vi "DUT_Handler_Simple_SoftFP.vi"(0 "reference in":refnum<class "DUT_Handler_Simple.lvclass">, 2 "Floating":bool, 5 "error in (no error)":errorcluster) -> (14 "reference out":refnum<class "DUT_Handler_Simple.lvclass">, 19 "error out":errorcluster)   [LabVIEW 2022 SP3, in "DUT_Handler_Simple.lvlib" / "DUT_Handler_Simple.lvclass"]
uses:
  DUT_Handler_Simple.lvclass
  Components/DUT_Handler_Base.lvlibp/EventData.ctl
  Components/ViPER.lvlibp/ViPER.lvclass
  C:/Projects/Medulla/ViPER/Examples/Flux_Capacitor_Tester/Components/ViPER.lvlibp/ViPER.lvclass
  Components/DUT_Handler_Base.lvlibp/DUT_Handler_Base.lvclass
panel:
  in  "Enable":bool
  in  "Load":bool
  out "event_data":T1={"Action"=enum."MoveIn", "SN"="", "BN"="", "DUT__ID"=0, "Message"="", "From"="", "To"=""}
  out "Enabled":bool
  in  "Move To":string
  in  "Move Out":bool
  in  "Move In":bool
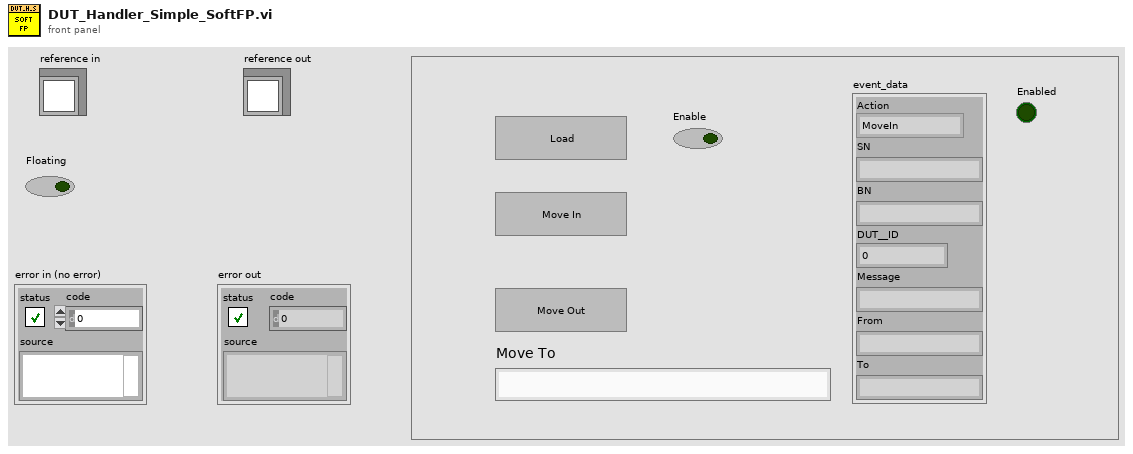
[diagram p1: front panel]
types:
  T1 = typedef "DUT_Handler_Base.lvlibp/DUT_Handler_Base.lvclass/EventData.ctl" = cluster{"Action":enum16{"Load", "Cancel", "MoveIn", "MoveOut", "Abort", "Msg", "Enabled", "Disabled", "Fault", "Shutdown"}, "SN":string, "BN":string, "DUT__ID":u32, "Message":string, "From":string, "To":string}
  T2 = enum32{"Invalid", "Standard", "Closed", "Hidden", "Minimized", "Maximized"}
  T3 = typedef "DUT_Handler_Simple.lvlib/DUT_Handler_Simple.lvclass/ObjectAttributes.ctl" = cluster{"Config":T4, "event_data":T1, "Enabled":bool, "Barcode_Reader":refnum<class "Barcode_Reader_Base.lvclass">}
  T4 = typedef "DUT_Handler_Simple.lvlib/DUT_Handler_Simple.lvclass/Config.ctl" = cluster{"default":string}
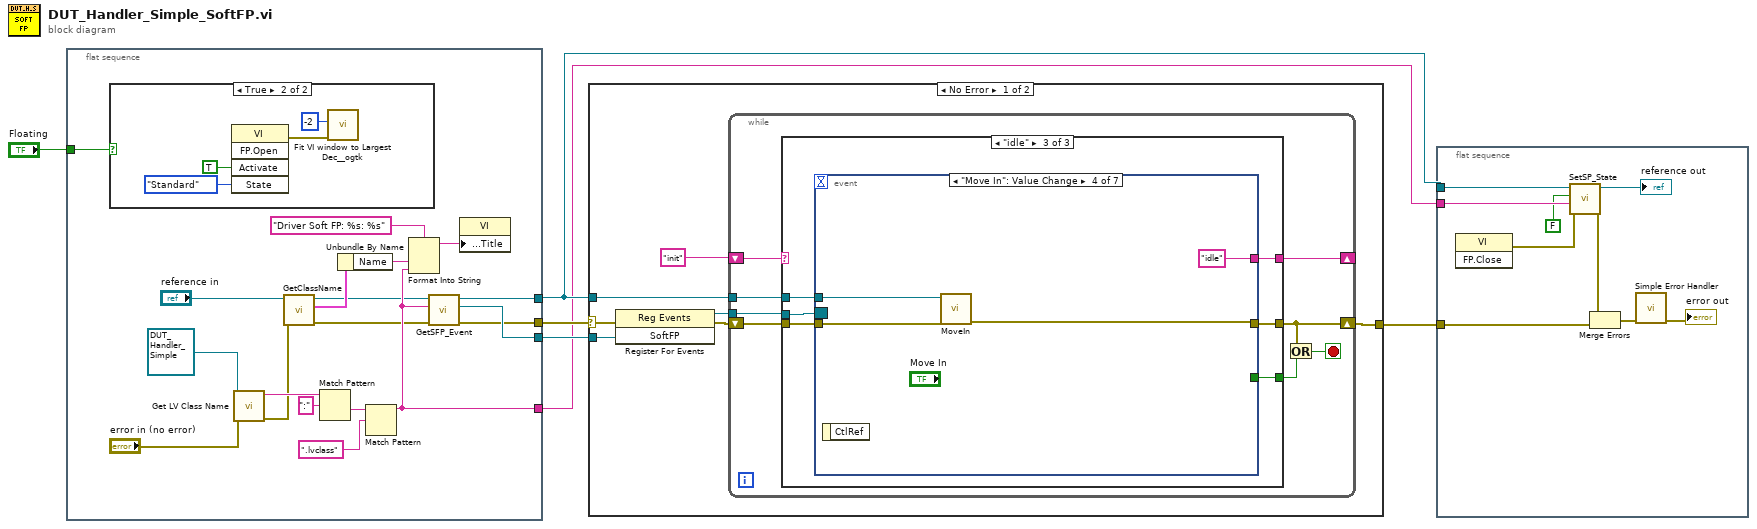
[diagram p0: block diagram]
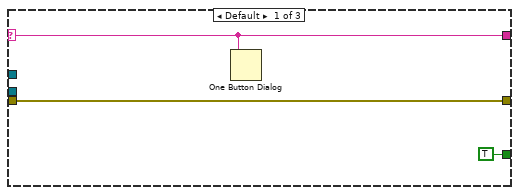
[diagram p3: hidden frame]
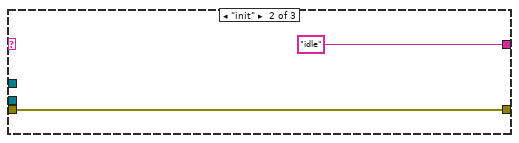
[diagram p4: hidden frame]
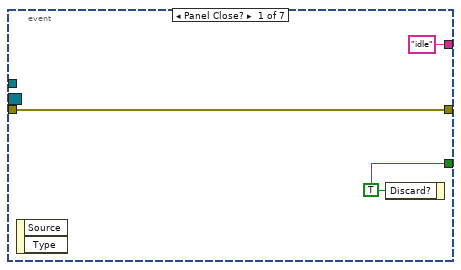
[diagram p5: hidden frame]
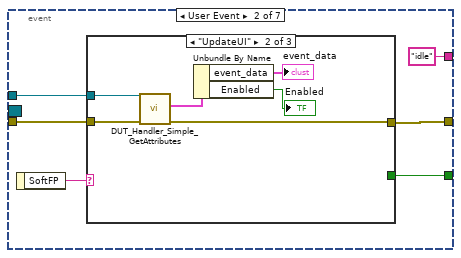
[diagram p6: hidden frame]
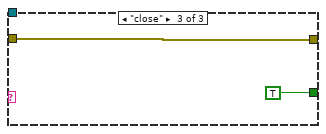
[diagram p8: hidden frame]
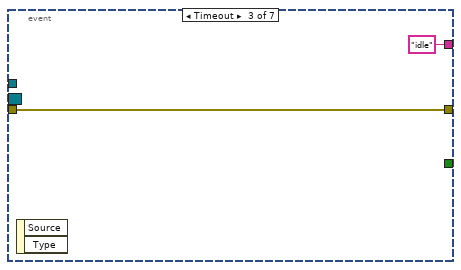
[diagram p9: hidden frame]
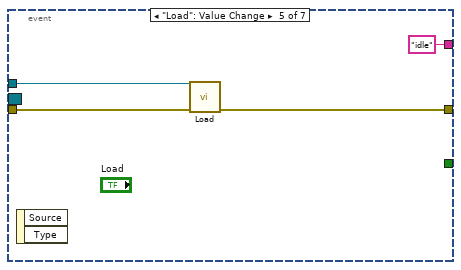
[diagram p10: hidden frame]
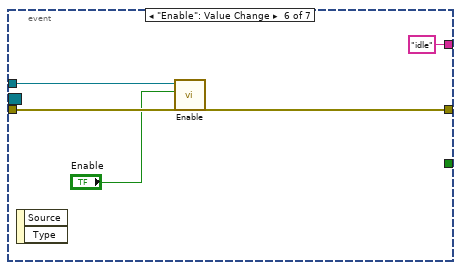
[diagram p11: hidden frame]
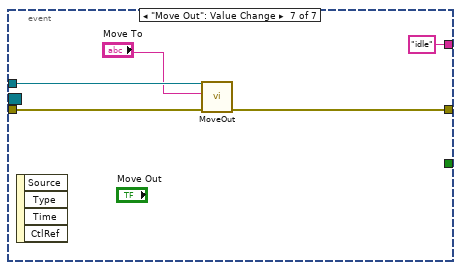
[diagram p12: hidden frame]
diagram:
  n1 = flat-sequence {
    tunnel: [w9] -> w6
    tunnel: [w8] -> w3
    tunnel: [w25] -> w4
    tunnel: [w15] -> w2
    tunnel: "Floating" -> [w7]
    frame #0 {
      n2 = case shown="True" w7 {
        frame False {
        }
        frame True {
          n3 = invoke class="VI" method="FP.Open"("Activate"=TRUE ("Activate?"), "State"=T2."Standard") -> (error out=w26:errorcluster)  [unwired: 3 in, 4 out]
          n4 = call <userlib>:"Fit VI window to Largest Dec__ogtk.vi"("error in (no error)"=w26, "border spacing (2 px)"=-2) -> ()  [unwired: 4 in, 2 out]
        }
      }
      n5 = call <vilib>:"Get LV Class Name.vi"("error in (no error)"="error in (no error)", "object"=refnum<class "DUT_Handler_Simple.lvclass"> refnum ("reference")) -> ("error out"=w14:errorcluster, "class name"=w20:string)  [unwired: 8 in]
      n6 = call "GetClassName.vi"("error in (no error)"=w14, "reference in"="reference in") -> ("error out"=w13:errorcluster, "Details"=w12:cluster{"Name":string, "Class":string}, "reference out"=w10:refnum<class "DUT_Handler_Simple.lvclass">)  [unwired: 7 in]
      n7 = Match Pattern(string=w20, regular expression=":") -> (after substring=w18:string)  [unwired: 1 in, 3 out]
      n8 = Unbundle By Name(w12) -> ("Name"=w22:string)
      n9 = Match Pattern(string=w18, regular expression=".lvclass") -> (before substring=w15:string)  [unwired: 1 in, 3 out]
      n10 = Format Into String(format string="Driver Soft FP: %s: %s", w22, w15) -> (resulting string=w24:string)  [unwired: 2 in, 1 out]
      n11 = call-dynamic "GetSFP_Event.vi"("error in (no error)"=w13, "Ancestor"=w15, "reference in"=w10) -> ("error out"=w9:errorcluster, "SoftFP"=w25:refnum<user-event>, "reference out"=w8:refnum<class "DUT_Handler_Simple.lvclass">)  [unwired: 6 in]
      n12 = property class="VI"("Front Panel.Title"=w24) -> ()  [unwired: 2 in, 2 out]
    }
  }
  n13 = case shown="No Error" w6 {
    selector: w6 -> [w34 w94]
    tunnel: [w30 w94] -> w5
    tunnel: w3 -> [w31 _]
    tunnel: w4 -> [w36 _]
    frame No Error {
      n14 = register-events(error in=w34, w36) -> (reference out=w35:refnum<event-registration>, error out=w33:errorcluster)  [unwired: 1 in]
      n15 = while {
        shift-right: [w41] -> w30
        shift-left: w33 -> [w44]
        tunnel: w35 -> [w43]
        tunnel: w31 -> [w42]
        shift-right: [w37] -> _
        shift-left: "init" -> [w38]
        stop <- w40 stop-if-true
        n16 = case shown="\"idle\"" w38 {
          selector: w38 -> [w45 _ _]
          tunnel: w44 -> [w46 w48 w55]
          tunnel: w43 -> [_ _ w54]
          tunnel: w42 -> [_ _ w53]
          tunnel: [w46 w48 w52] -> w41
          tunnel: [TRUE ("Discard?") _ w51] -> w39
          tunnel: [w45 "idle" w50] -> w37
          frame Default {
            n17 = One Button Dialog(message=w45) -> ()  [unwired: 1 in, 1 out]
          }
          frame "init" {
          }
          frame "idle" {
            n18 = event shown="[3] \"Move In\": Value Change" {
              selector: w54 -> [_ _ _ _ _ _ _]
              dyn-events: _ -> [_ _ _ _ _ _ _]
              timeout: _ -> [_ _ _ _ _ _ _]
              tunnel: w55 -> [w58 w64 w75 w79 w83 w87 w93]
              tunnel: [w58 w62 w75 w77 w81 w86 w92] -> w52
              tunnel: [w57 w61 _ _ _ _ _] -> w51
              tunnel: w53 -> [_ w59 _ w78 w82 w85 w91]
              tunnel: ["idle" "idle" "idle" "idle" "idle" "idle" "idle"] -> w50
              event Panel Close? {
                w57 = TRUE ("Discard?")
                n19 = event-data() -> ()  [unwired: 1 in, 2 out]
                n20 = event-data("Discard?"=w57) -> ()  [unwired: 1 in, 1 out]
              }
              event User Event {
                n21 = event-data() -> ("SoftFP"=w63:string)  [unwired: 1 in]
                n22 = case shown="\"UpdateUI\"" w63 {
                  tunnel: w64 -> [w65 w71 w73]
                  tunnel: [w65 w70 w73] -> w62
                  tunnel: [_ _ TRUE ("Discard?")] -> w61
                  tunnel: w59 -> [_ w69 _]
                  frame Default {
                  }
                  frame "UpdateUI" {
                    n23 = call "DUT_Handler_Simple_GetAttributes.vi"("error in (no error)"=w71, "reference in"=w69) -> ("error out"=w70:errorcluster, "Data"=w68:T3)  [unwired: 6 in, 2 out]
                    n24 = Unbundle By Name(w68) -> ("event_data"=→"event_data":T1, "Enabled"=→"Enabled":bool)
                  }
                  frame "close" {
                  }
                }
              }
              event Timeout {
                n25 = event-data() -> ()  [unwired: 1 in, 2 out]
              }
              event "Move In": Value Change {
                n26 = event-data() -> ()  [unwired: 1 in, 1 out]
                n27 = call-dynamic "MoveIn.vi"("error in (no error)"=w79, "reference in"=w78) -> ("error out"=w77:errorcluster)  [unwired: 7 in, 2 out]
              }
              event "Load": Value Change {
                n28 = event-data() -> ()  [unwired: 1 in, 2 out]
                n29 = call-dynamic "Load.vi"("error in (no error)"=w83, "reference in"=w82) -> ("error out"=w81:errorcluster)  [unwired: 7 in, 2 out]
              }
              event "Enable": Value Change {
                n30 = event-data() -> ()  [unwired: 1 in, 2 out]
                n31 = call-dynamic "Enable.vi"("error in (no error)"=w87, "Enable?"="Enable", "reference in"=w85) -> ("error out"=w86:errorcluster)  [unwired: 7 in, 1 out]
              }
              event "Move Out": Value Change {
                n32 = event-data() -> ()  [unwired: 1 in, 4 out]
                n33 = call-dynamic "MoveOut.vi"("error in (no error)"=w93, "Destination"="Move To", "reference in"=w91) -> ("error out"=w92:errorcluster)  [unwired: 7 in, 1 out]
              }
            }
          }
        }
        n34 = Or(x=w41, y=w39) -> (x .or. y?=w40:bool)
      }
    }
    frame Error {
    }
  }
  n35 = flat-sequence {
    tunnel: w5 -> [w101]
    tunnel: w3 -> [w96]
    tunnel: w2 -> [w98]
    frame #0 {
      n36 = invoke class="VI" method="FP.Close"() -> (error out=w100:errorcluster)  [unwired: 3 in, 2 out]
      n37 = call "SetSP_State.vi"("error in (no error)"=w100, "Ancestor"=w98, "SP Open"=FALSE, "reference in"=w96) -> ("error out"=w99:errorcluster, "reference out"=→"reference out":refnum<class "DUT_Handler_Simple.lvclass">)  [unwired: 6 in]
      n38 = Merge Errors(w99, w101) -> (w103:errorcluster)
      n39 = call <vilib>:"Simple Error Handler.vi"("error in (no error)"=w103) -> ("error out"=→"error out":errorcluster)  [unwired: 4 in, 4 out]
    }
  }
